vi "Guardians Status Check.vi"(8 "error in (no error)":errorcluster, 11 "Guardian in":refnum<class "Guardian.lvclass">) -> (0 "error out":errorcluster, 3 "Guardian out":refnum<class "Guardian.lvclass">)   [LabVIEW 2026, in "TALOS.lvlib" / "Guardian.lvlib" / "Guardian.lvclass"]
doc: "This VI checks the status of all the Guardians present in the network.\nIt opens all the AEgIS Shared Variables (ASV) Guadian_Health_*, and for all of them it confronts the timestamp of the Last Poke with now: if the delta time, for one (or more) of them, is bigger than the parameter Guardian_Check_tau_s, the Guardian_Health_ ASV of that specific Guardian is marked Alive=False and a Guardian Died Recheck? is scheduled (where basically the Alive status is checked again: if the appropriate Guardian has set Alive back to True, nothing is done, otherwise it means it's really dead, and ABORT is initiated).\nConcurrently, it also check the status of its own Guardian_Health_ ASV, and in case was set Alive=False by any other Guardian. it restores it to True. It also update the list of the Guardian to be displayed on the screen."
uses:
  Guardian.lvclass
  C:/LabVIEW Code/TALOS/talos/Ancestor/Ancestor/Ancestor.lvclass
  C:/LabVIEW Code/TALOS/builds/Actor Framework PPL/Actor Framework.lvlibp/1abvi3w/vi.lib/ActorFramework/Actor/Actor.lvclass
  Ancestor/Ancestor/Ancestor.lvclass/Ancestor.ctl
  Classes/Speedometer/Speedometer.lvclass/Speedometer.ctl
  Guardian.lvclass/Guardian.ctl
  Guardian Messages/Guardian Died Recheck Msg/Guardian Died Recheck Msg.lvclass/Guardian Died Recheck Msg.ctl
  Guardian Messages/Message to Other Guardian Msg/Message to Other Guardian Msg.lvclass/Message to Other Guardian Msg.ctl
  Ancestor/Ancestor/Read ID.vi
  Support VIs/Generate Error.vi
  <vilib>/Utility/High Resolution Relative Seconds.vi
  Guardian Messages/Guardian Died Recheck Msg/Write ID.vi
  FGV/Error Memory/Get Error Description.vi
  Support VIs/Get PC name.vi
  Support VIs/Get Class Name.vi
  FGV/Error Memory/Error Memory Core.vi
  <vilib>/AdvancedString/Delimited String to 1D String Array.vi
  <vilib>/AdvancedString/Delimited String to 1D String Array (string).vi
  Support VIs/Circus Root Path.vi
  FGV/Error Memory/Error Crt Lvl checker.vi
  FGV/Error Memory/Error Memory Core.vi/40c8088d-b597-4017-91af-faa98e00292e.vi
  FGV/Error Memory/Error Memory Core.vi/d4a3ab98-063c-4e44-b43d-fbdcfe6c2be2.vi
  Guardian Messages/Guardian Died Recheck Msg/Guardian Died Recheck Msg.lvclass
  C:/LabVIEW Code/TALOS/builds/Actor Framework PPL/Actor Framework.lvlibp/1abvi3w/vi.lib/ActorFramework/Message/Message.lvclass
  Support VIs/Global Memory.vi
  <vilib>/Utility/LVClass/Get LV Class Name.vi
  Support VIs/Is in Packed Library.vi
  Support VIs/TALOS Root path.vi
  Support VIs/Read CSV worksheet.vi
  Support VIs/Global Constants.vi
  <vilib>/Utility/error.llb/General Error Handler.vi
  <vilib>/Utility/config.llb/Open Config Data.vi
  <vilib>/Utility/config.llb/Get Section Names.vi
  <vilib>/Utility/config.llb/Get Key Names.vi
  <vilib>/Utility/config.llb/Read Key.vi
  <vilib>/Utility/config.llb/Read Key (String).vi
  <vilib>/Utility/config.llb/Close Config Data.vi
  builds/Actor Framework PPL/Actor Framework.lvlibp/1abvi3w/vi.lib/ActorFramework/Time-Delayed Send Message/Time-Delayed Send Message.vi
  Support VIs/Error Log.vi
  builds/Actor Framework PPL/Actor Framework.lvlibp/1abvi3w/vi.lib/ActorFramework/Message Enqueuer/Enqueue.vi
  Support VIs/System Log.vi
  Ancestor/Ancestor/Ancestor.lvclass
  <vilib>/Comparison/Equal/Equal Functor/Equal Functor.lvclass
  Classes/Speedometer/Speedometer.lvclass
  Guardian Messages/Message to Other Guardian Msg/Message to Other Guardian Msg.lvclass
  Classes/Guardian List/Guardian List.lvclass
  builds/Actor Framework PPL/Actor Framework.lvlibp/1abvi3w/vi.lib/ActorFramework/Actor/Actor.lvclass
  TALOS.lvlib
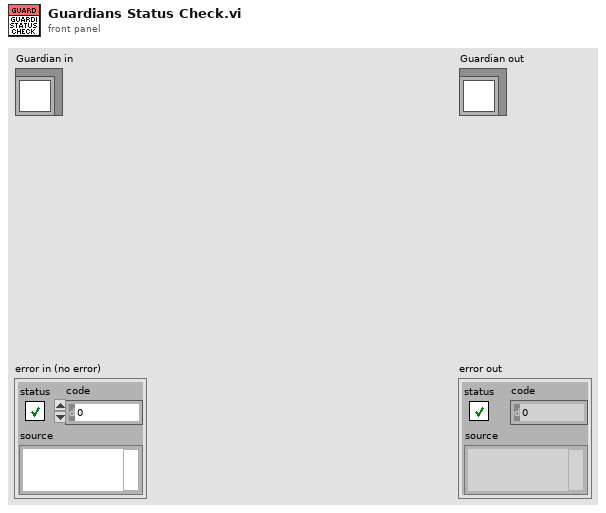
[diagram p1: front panel]
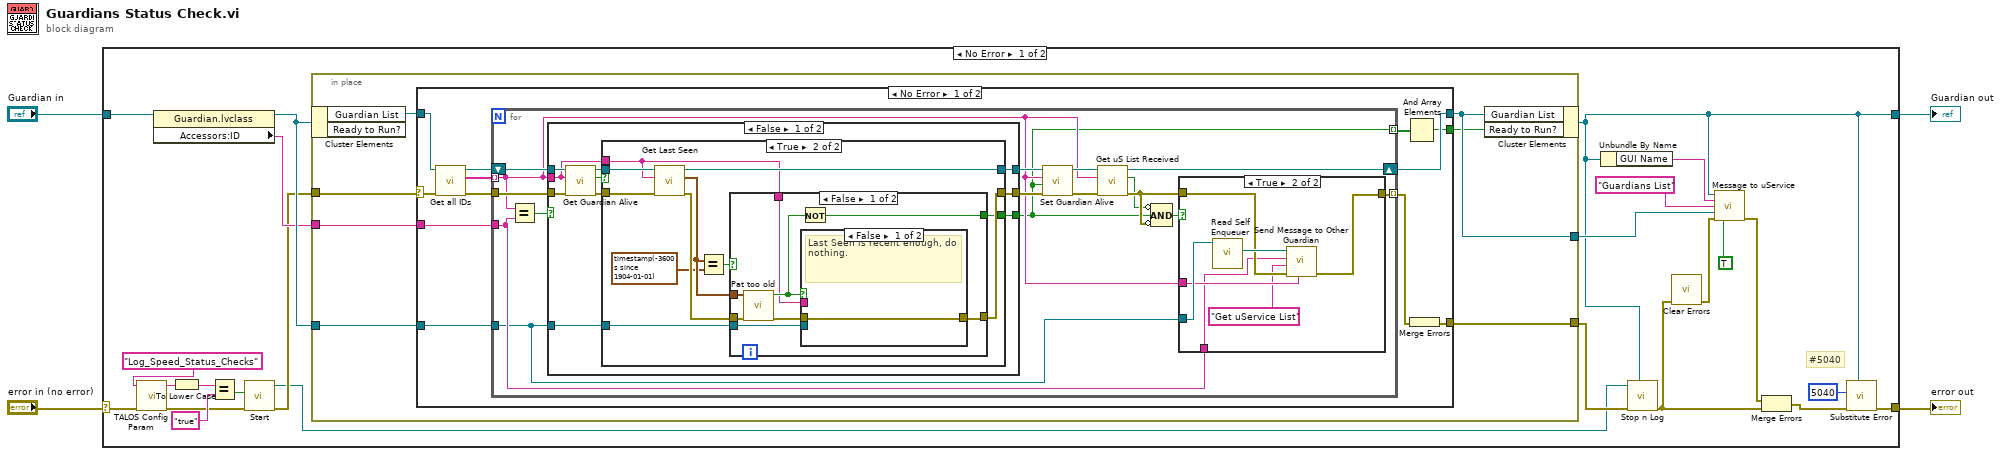
[diagram p0: block diagram]
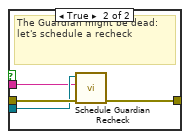
[diagram p3: hidden frame]
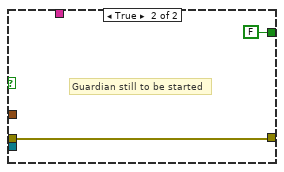
[diagram p4: hidden frame]
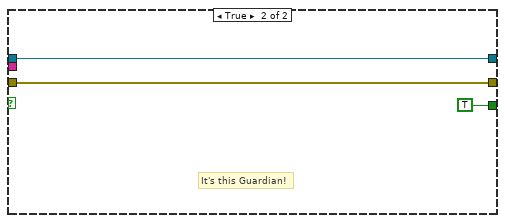
[diagram p5: hidden frame]
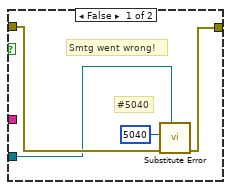
[diagram p6: hidden frame]
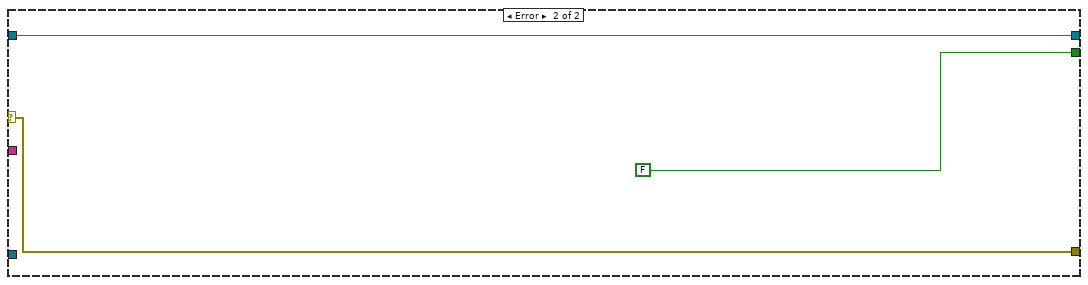
[diagram p7: hidden frame]
diagram:
  n1 = case shown="No Error" "error in (no error)" {
    selector: "error in (no error)" -> [w11 w121]
    tunnel: [w6 w121] -> w2
    tunnel: [w5 w120] -> w1
    tunnel: "Guardian in" -> [w28 w120]
    frame No Error {
      # "#5040"
      n2 = call "TALOS Config Param.vi"("error in (no error)"=w11, "Parameter Name"="Log_Speed_Status_Checks") -> ("error out"=w10:errorcluster, "Output"=w15:string)  [unwired: 8 in]
      n3 = property class="Guardian.lvclass"(reference=w28) -> (reference out=w22:refnum<class "Guardian.lvclass">, "Accessors:ID"=w21:string)  [unwired: 1 in, 1 out]
      n4 = To Lower Case(string=w15) -> (all lower case string=w14:string)
      n5 = Equal?(x=w14, y="true") -> (x = y?=w9:bool)
      n6 = call "Start.vi"("error in (no error)"=w10, "Active?"=w9) -> ("error out"=w20:errorcluster, "Speedometer out"=w18:refnum<class "Speedometer.lvclass">)  [unwired: 8 in]
      n7 = in-place "In Place Element Structure" {
        in-place-border: [w35] -> w19
        in-place-border: w22 -> [w31]
        in-place-border: w20 -> [w34]
        in-place-border: [w32] -> w26
        in-place-border: w21 -> [w29]
        n8 = in-place-cluster #1(w22) -> ("Guardian List"=w33:refnum<class "Guardian List.lvclass">)  [unwired: 1 out]
        n9 = case shown="No Error" w34 {
          selector: w34 -> [w44 w119]
          tunnel: [w47 w119] -> w35
          tunnel: w33 -> [w43 w118]
          tunnel: [w42 w118] -> w32
          tunnel: w31 -> [w41 _]
          tunnel: [w37 FALSE] -> w30
          tunnel: w29 -> [w36 _]
          frame No Error {
            n10 = call-dynamic "Get all IDs.vi"("error in (no error)"=w44, "Guardian List in"=w43) -> ("error out"=w39:errorcluster, "All IDs"=w46:string[], "Guardian List out"=w45:refnum<class "Guardian List.lvclass">)  [unwired: 7 in]
            n11 = for {
              tunnel: w46 -> [w53] mode=indexing
              shift-right: [w54] -> w42
              shift-left: w45 -> [w62]
              tunnel: w41 -> [w48]
              tunnel: [w51] -> w40 mode=indexing
              tunnel: w39 -> [w59]
              tunnel: [w49] -> w38 mode=indexing
              tunnel: w36 -> [w52]
              n12 = Equal?(x=w53, y=w52) -> (x = y?=w58:bool)
              n13 = case shown="False" w58 {
                tunnel: w62 -> [w66 w104]
                tunnel: [w73 w104] -> w61
                tunnel: [w72 w103] -> w60
                tunnel: w48 -> [w71 _]
                tunnel: w53 -> [w65 _]
                tunnel: w59 -> [w68 w103]
                tunnel: [w70 TRUE] -> w49
                frame False {
                  n14 = call-dynamic "Get Guardian Alive.vi"("error in (no error)"=w68, "ID"=w65, "Guardian List in"=w66) -> ("error out"=w69:errorcluster, "Alive"=w64:bool, "Guardian List out"=w67:refnum<class "Guardian List.lvclass">)  [unwired: 6 in]
                  n15 = case shown="True" w64 {
                    selector: w64 -> [w74 _]
                    tunnel: [w76 w87] -> w73
                    tunnel: [w75 w85] -> w72
                    tunnel: w71 -> [_ w84]
                    tunnel: [w74 w83] -> w70
                    tunnel: w69 -> [w75 w79]
                    tunnel: w67 -> [w76 w78]
                    tunnel: w65 -> [_ w77]
                    frame False {
                      # "Guardian not alive, do not check its status (it could give an infinite Error 5004 (GD down)"
                    }
                    frame True {
                      n16 = call-dynamic "Get Last Seen.vi"("error in (no error)"=w79, "ID"=w77, "Guardian List in"=w78) -> ("error out"=w86:errorcluster, "Last Poke"=w81:timestamp, "Guardian List out"=w87:refnum<class "Guardian List.lvclass">)  [unwired: 6 in]
                      n17 = Equal?(x=w81, y=timestamp(-3600 s since 1904-01-01)) -> (x = y?=w82:bool)
                      n18 = case shown="False" w82 {
                        tunnel: w81 -> [w93 _]
                        tunnel: w86 -> [w92 w102]
                        tunnel: [w91 w102] -> w85
                        tunnel: w84 -> [w90 _]
                        tunnel: w77 -> [w89 _]
                        tunnel: [w88 FALSE] -> w83
                        frame False {
                          n19 = call "Pat too old.vi"("error in (no error)"=w92, "Last Seen"=w93) -> ("error out"=w94:errorcluster, "Too old?"=w95:bool)  [unwired: 8 in]
                          n20 = Not(x=w95) -> (.not. x?=w88:bool)
                          n21 = case shown="False" w95 {
                            tunnel: w94 -> [w96 w99]
                            tunnel: [w96 w100] -> w91
                            tunnel: w90 -> [_ w98]
                            tunnel: w89 -> [_ w97]
                            frame False {
                              # "Last Seen is recent enough, do nothing."
                            }
                            frame True {
                              # "The Guardian might be dead: let's schedule a recheck"
                              n22 = call "Schedule Guardian Recheck.vi"("error in (no error)"=w99, "Guardian ID"=w97, "Guardian in"=w98) -> ("error out"=w100:errorcluster)  [unwired: 7 in, 1 out]
                            }
                          }
                        }
                        frame True {
                          # "Guardian still to be started"
                        }
                      }
                    }
                  }
                }
                frame True {
                  # "It's this Guardian!"
                }
              }
              n23 = call-dynamic "Set Guardian Alive.vi"("error in (no error)"=w60, "Alive"=w49, "ID"=w53, "Guardian List in"=w61) -> ("error out"=w56:errorcluster, "Guardian List out"=w57:refnum<class "Guardian List.lvclass">)  [unwired: 6 in]
              n24 = call-dynamic "Get uS List Received.vi"("error in (no error)"=w56, "ID"=w53, "Guardian List in"=w57) -> ("error out"=w63:errorcluster, "uS List Received"=w55:bool, "Guardian List out"=w54:refnum<class "Guardian List.lvclass">)  [unwired: 6 in]
              n25 = Compound Arithmetic op=AND(invert w55, w49, invert w63) -> (w50:bool)
              n26 = case shown="True" w50 {
                tunnel: w48 -> [w107 w116]
                tunnel: w63 -> [w109 w114]
                tunnel: w53 -> [_ w113]
                tunnel: w52 -> [_ w111]
                tunnel: [w108 w110] -> w51
                frame False {
                  # "Smtg went wrong!"
                  # "#5040"
                  n27 = call "Substitute Error.vi"("LabVIEW Object"=w107, "error in (no error)"=w109, "Error Code"=5040) -> ("error out"=w108:errorcluster)  [unwired: 8 in]
                }
                frame True {
                  n28 = call "Read Self Enqueuer.vi"("Actor"=w116) -> ("Self Enqueuer"=w115:refnum<class "Message Enqueuer.lvclass">)  [unwired: 10 in]
                  n29 = call "Send Message to Other Guardian.vi"("Guardian ID"=w113, "error in (no error)"=w114, "Message"="Get uService List", "Data"=w111, "Message Enqueuer"=w115) -> ("error out"=w110:errorcluster)  [unwired: 5 in, 1 out]
                }
              }
            }
            n30 = And Array Elements(Boolean array=w38) -> (logical AND=w37:bool)
            n31 = Merge Errors(w40) -> (w47:errorcluster)
          }
          frame Error {
          }
        }
        n32 = in-place-cluster #1("Guardian List"=w32, "Ready to Run?"=w30) -> (w5:refnum<class "Guardian.lvclass">)
      }
      n33 = Unbundle By Name(w5) -> ("GUI Name"=w27:string)
      n34 = call "Stop n Log.vi"("Object in"=w5, "error in (no error)"=w19, "Speedometer in"=w18) -> ("error out"=w17:errorcluster)  [unwired: 8 in]
      n35 = call <vilib>:"Clear Errors.vi"("error in (no error)"=w17) -> ("error out"=w16:errorcluster)  [unwired: 5 in, 1 out]
      n36 = call "Message to uService.vi"("Guardian in"=w5, "uService ID"=w27, "Message"="Guardians List", "Data"=w26, "error in (no error)"=w16, "Locale?"=TRUE) -> ("error out"=w24:errorcluster)  [unwired: 8 in, 1 out]
      n37 = Merge Errors(w24, w17) -> (w7:errorcluster)
      n38 = call "Substitute Error.vi"("LabVIEW Object"=w5, "error in (no error)"=w7, "Error Code"=5040) -> ("error out"=w6:errorcluster)  [unwired: 8 in]
    }
    frame Error {
    }
  }
  "error out" <- w2
  "Guardian out" <- w1
